vi "Array to Merge Signal.vi"() -> ()   [LabVIEW 2023]
panel:
  in  "Loop Number":i32
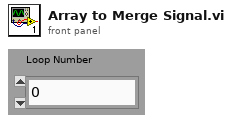
[diagram p1: front panel]
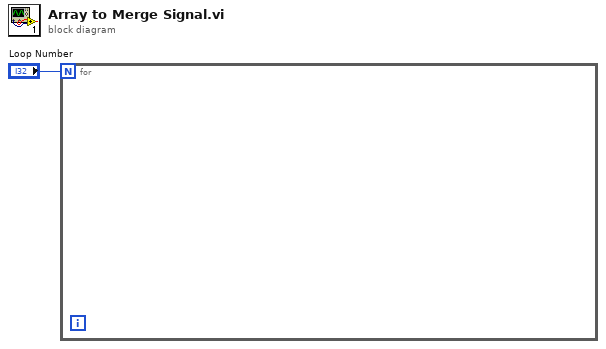
[diagram p0: block diagram]
diagram:
  n1 = for {
    N: "Loop Number" -> [_]
  }
